vi "Sim flow temp pressure.vi"(10 "Offset":dbl, 11 "Spectral Amplitude":dbl) -> (3 "Array":dbl[][](array[numeric]))   [LabVIEW 2018]
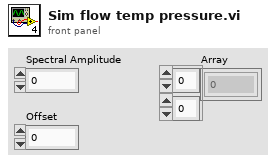
[diagram p1: front panel]
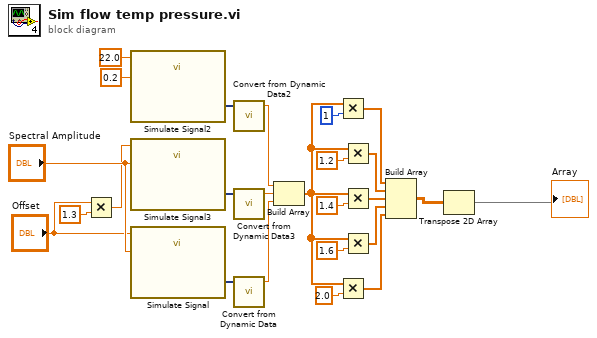
[diagram p0: block diagram]
diagram:
  n1 = Multiply(x="Offset", y=1.3) -> (x*y=w13:dbl)
  n2 = call "Simulate Signal2"("Offset"=22.0, "Spectral amplitude"=0.2) -> ("DC Temperature Signal"=w9:dynamicdata)  [unwired: 12 in, 1 out]
  n3 = call "Simulate Signal3"("Offset"=w13, "Spectral amplitude"="Spectral Amplitude") -> ("DC Pressure Signal"=w8:dynamicdata)  [unwired: 12 in, 1 out]
  n4 = call "Simulate Signal"("Offset"="Offset", "Spectral amplitude"="Spectral Amplitude") -> ("DC Flowrate Signal"=w10:dynamicdata)  [unwired: 12 in, 1 out]
  n5 = call "Convert from Dynamic Data2"("Dynamic Data Type"=w9) -> ("Scalar"=w15:dbl)  [unwired: 3 in]
  n6 = call "Convert from Dynamic Data3"("Dynamic Data Type"=w8) -> ("Scalar"=w16:dbl)  [unwired: 3 in]
  n7 = call "Convert from Dynamic Data"("Dynamic Data Type"=w10) -> ("Scalar"=w17:dbl)  [unwired: 3 in]
  n8 = Build Array(w15, w16, w17) -> (w22:dbl[])
  n9 = Multiply(x=w22, y=1) -> (x*y=w19:dbl[])
  n10 = Multiply(x=w22, y=2.0) -> (x*y=w5:dbl[])
  n11 = Multiply(x=w22, y=1.2) -> (x*y=w21:dbl[])
  n12 = Multiply(x=w22, y=1.4) -> (x*y=w7:dbl[])
  n13 = Multiply(x=w22, y=1.6) -> (x*y=w6:dbl[])
  n14 = Build Array(w19, w21, w7, w6, w5) -> (w2:dbl[][])
  n15 = Transpose 2D Array(2D array=w2) -> (transposed array=→"Array":dbl[][])
